vi "Add or Subtract Fixturing ROI.vi"(8 "error control":errorcluster, 9 "ROI in":T2, 10 "Fixturing ROI":i32[](array[numeric]), 11 "Enum":T1(ring)) -> (0 "error indicator":errorcluster, 3 "ROI out":T2)   [LabVIEW 2020]
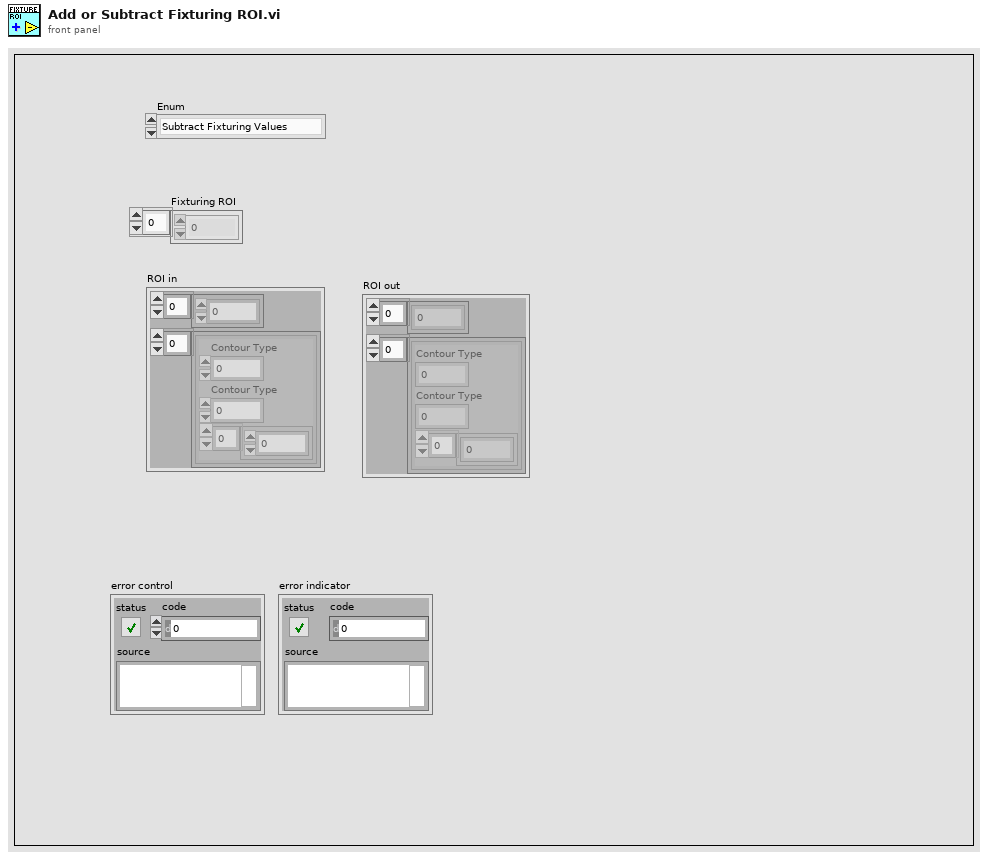
[diagram p1: front panel]
types:
  T1 = enum16{"Subtract Fixturing Values ", "Add Fixturing Values"}
  T2 = cluster{i32[], cluster{"Contour Type":u32, "Contour Type":i32, i32[]}[]}
  T3 = cluster{"Contour Type":u32, "Contour Type":i32, i32[]}[]
  T4 = cluster{"Contour Type":u32, "Contour Type":i32, i32[]}
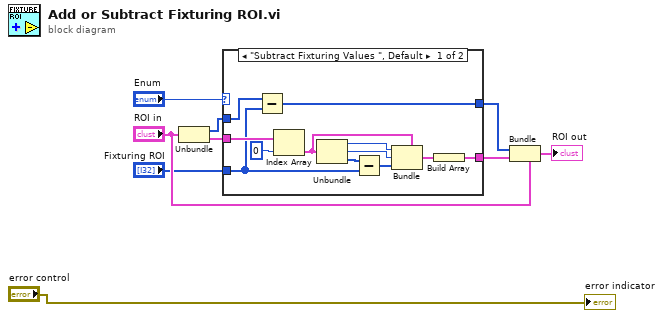
[diagram p0: block diagram]
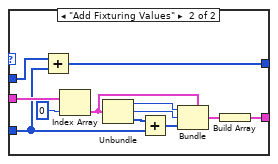
[diagram p2: hidden frame]
diagram:
  n1 = Unbundle("ROI in") -> (w4:i32[], w9:T3)
  n2 = case shown="\"Subtract Fixturing Values \", Default" "Enum" {
    tunnel: w9 -> [w12 w33]
    tunnel: [w13 w26] -> w7
    tunnel: [w14 w25] -> w5
    tunnel: w4 -> [w11 w24]
    tunnel: "Fixturing ROI" -> [w10 w22]
    frame "Subtract Fixturing Values ", Default {
      n3 = Subtract(x=w11, y=w10) -> (x-y=w14:i32[])
      n4 = Index Array(array=w12, index=0) -> (element=w20:T4)
      n5 = Unbundle(w20) -> ("Contour Type"=w17:u32, "Contour Type"=w18:i32, w15:i32[])
      n6 = Subtract(x=w15, y=w10) -> (x-y=w19:i32[])
      n7 = Bundle(cluster=w20, "Contour Type"=w17, "Contour Type"=w18, w19) -> (w16:T4)
      n8 = Build Array(w16) -> (w13:T3)
    }
    frame "Add Fixturing Values" {
      n9 = Add(x=w24, y=w22) -> (x+y=w25:i32[])
      n10 = Index Array(array=w33, index=0) -> (element=w31:T4)
      n11 = Unbundle(w31) -> ("Contour Type"=w28:u32, "Contour Type"=w29:i32, w23:i32[])
      n12 = Add(x=w23, y=w22) -> (x+y=w30:i32[])
      n13 = Bundle(cluster=w31, "Contour Type"=w28, "Contour Type"=w29, w30) -> (w27:T4)
      n14 = Build Array(w27) -> (w26:T3)
    }
  }
  n15 = Bundle(cluster="ROI in", w5, w7) -> (→"ROI out":T2)
  "error indicator" <- "error control"
